vi "Read pos_est_x.vi"(8 "error in (no error)":errorcluster, 11 "Object in":refnum<class "Object.lvclass">) -> (0 "error out":errorcluster, 2 "pos_est_x":dbl, 3 "Object out":refnum<class "Object.lvclass">)   [LabVIEW 2023, in "Object.lvclass"]
uses:
  Object.lvclass
  Object.lvclass/Object.ctl
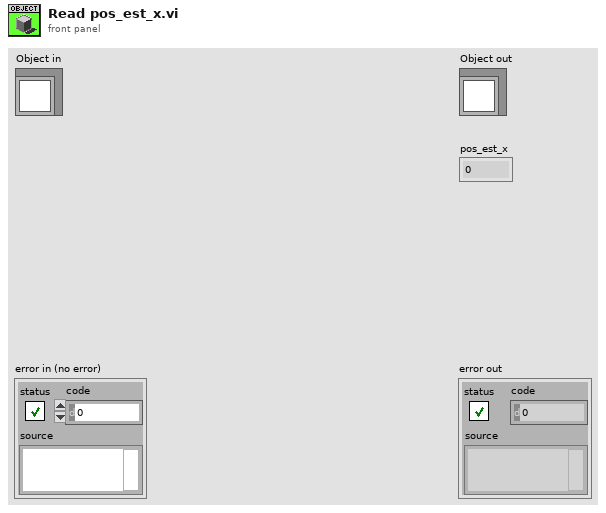
[diagram p1: front panel]
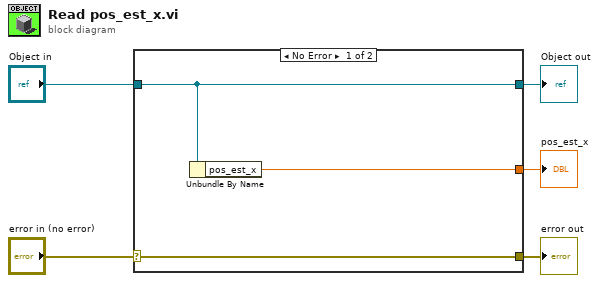
[diagram p0: block diagram]
diagram:
  n1 = case shown="No Error" "error in (no error)" {
    selector: "error in (no error)" -> [w8 w9]
    tunnel: [w8 w9] -> w4
    tunnel: [w7 w10] -> w2
    tunnel: "Object in" -> [w7 w10]
    tunnel: [w6 _] -> w1
    frame No Error {
      n2 = Unbundle By Name(w7) -> ("pos_est_x"=w6:dbl)
    }
    frame Error {
    }
  }
  "error out" <- w4
  "Object out" <- w2
  "pos_est_x" <- w1
